vi "SLSC_Determine_Resource.vi"(10 "SLSC Item":string, 11 "SLSC Module Name":string) -> (2 "Resource":string)   [LabVIEW 2015, in "SLSC Module Template Engine.lvlib"]
uses:
  SLSC Module Template Engine.lvlib
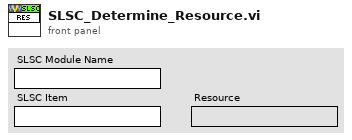
[diagram p1: front panel]
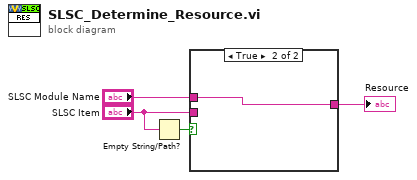
[diagram p0: block diagram]
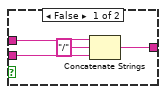
[diagram p2: hidden frame]
diagram:
  n1 = Empty String/Path?(string/path="SLSC Item") -> (empty?=w1:bool)
  n2 = case shown="True" w1 {
    tunnel: [w8 w9] -> w4
    tunnel: "SLSC Module Name" -> [w6 w9]
    tunnel: "SLSC Item" -> [w5 _]
    frame False {
      n3 = Concatenate Strings(w6, "/", w5) -> (w8:string)
    }
    frame True {
    }
  }
  "Resource" <- w4
